vi "Wavelength Meter Control Panel (No Objects).vi"(8 "error in (no error)":errorcluster) -> (0 "error out":errorcluster)   [LabVIEW 2012]
doc: "(Dynamic) A user-level application that simulates the physical front panel of the Instrument. Provide the user with buttons to manually control features of the instrument, and provide indicators of its current state."
uses:
  HighFinesse WS5/Variable Typedefs.llb/Exposure Mode.ctl
  HighFinesse WS5/Control typedefs.llb/Measurement Mode.ctl
  HighFinesse WS5/HighFinesse WS5.lvlib
panel:
  in  "Cluster In":T3={"Exp Range Min"=0, "Exp Range Max"=0, "exposure mode"=enum."manual", "operation (meas. mode)"=enum."Measurement mode", "Exposure (ms)"=0, "Quiet Errors?"=FALSE, "Error Status"={"status"=FALSE, "code"=0, "source"=""}}
  out "Ready":bool
  out "Exposure (ms)":u16
  in  "Exposure Mode":T1
  in  "stop":bool
  in  "Read":bool
  in  "Set Exposure (ms)":u16
  out "Wavelength":dbl
  in  "Copy Actual to set":bool
  in  "Populate Fields with member data":bool
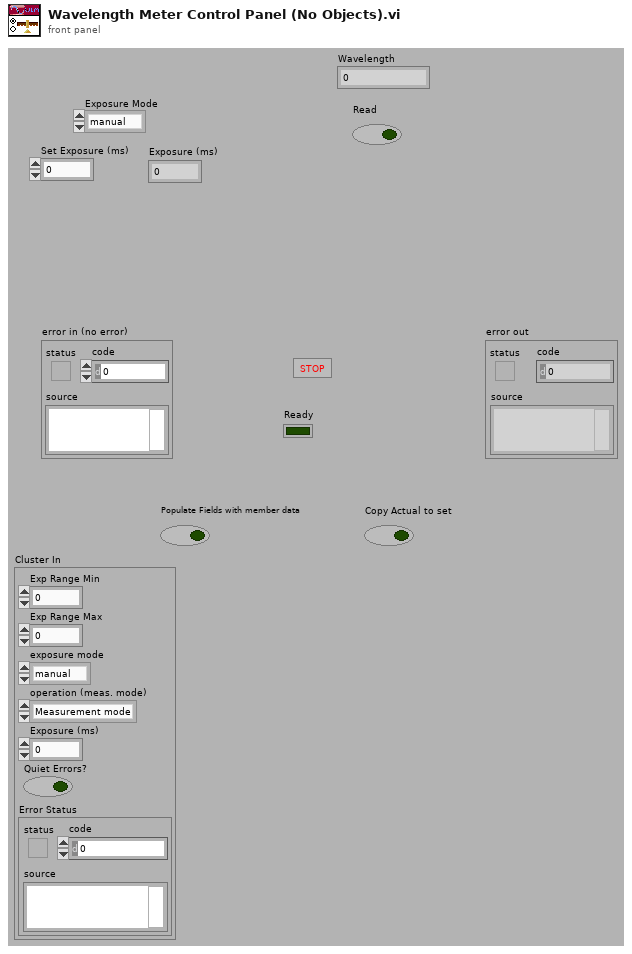
[diagram p1: front panel]
types:
  T1 = typedef "HighFinesse WS5.lvlib/Exposure Mode.ctl" = enum16{"manual", "automatic"}
  T2 = typedef "HighFinesse WS5.lvlib/Measurement Mode.ctl" = enum16{"Measurement off", "Adjustment mode", "Measurement mode"}
  T3 = cluster{"Exp Range Min":u32, "Exp Range Max":u32, "exposure mode":T1, "operation (meas. mode)":T2, "Exposure (ms)":u16, "Quiet Errors?":bool, "Error Status":errorcluster}
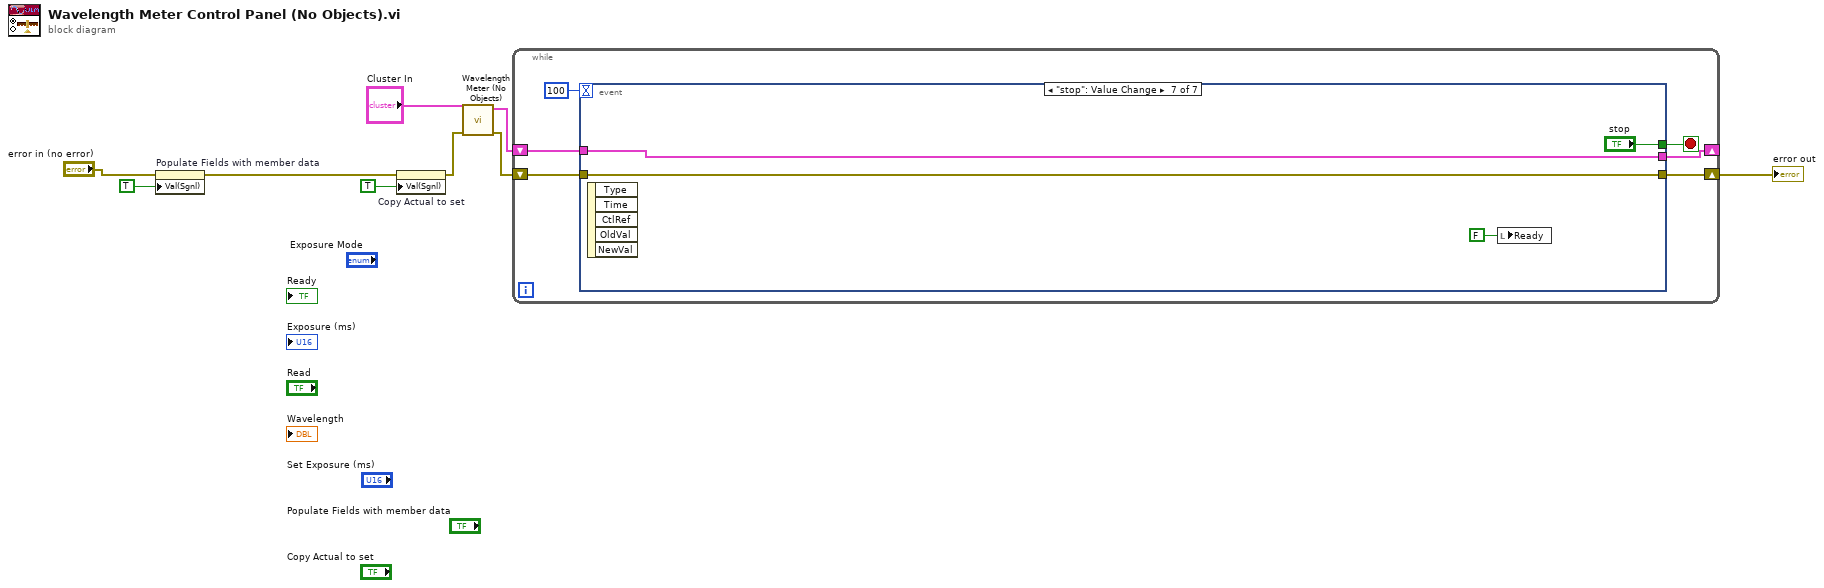
[diagram p0: block diagram]
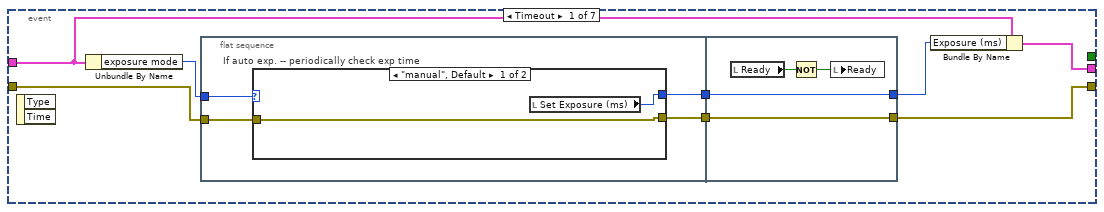
[diagram p2: hidden frame]
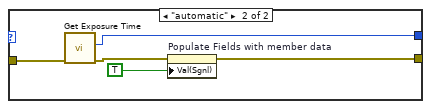
[diagram p3: hidden frame]
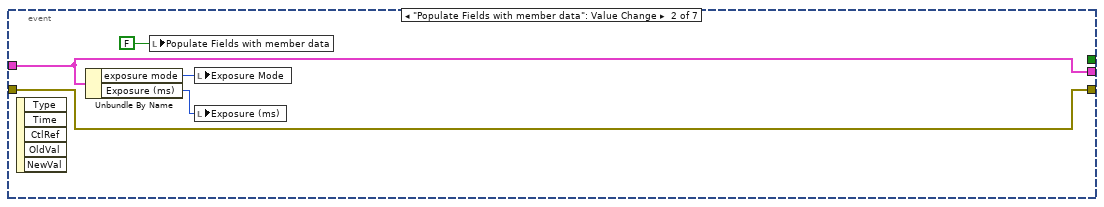
[diagram p4: hidden frame]
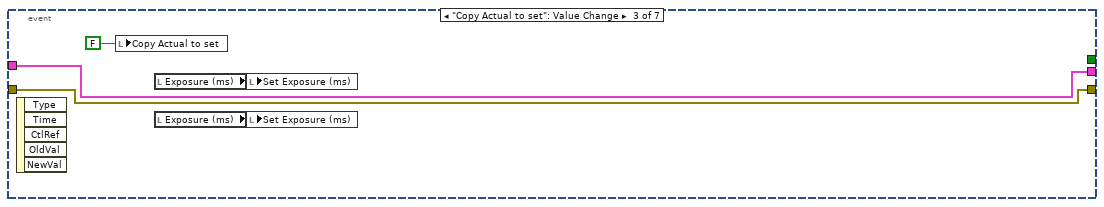
[diagram p5: hidden frame]
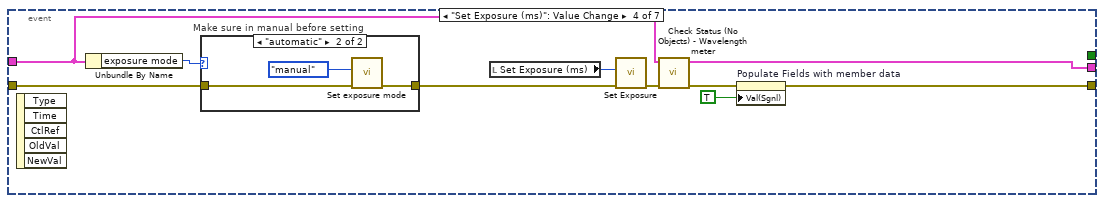
[diagram p6: hidden frame]
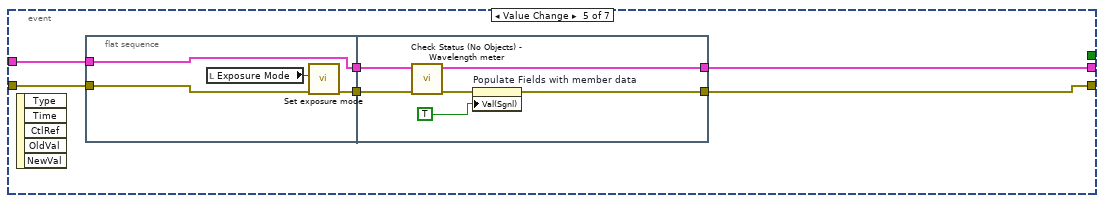
[diagram p8: hidden frame]
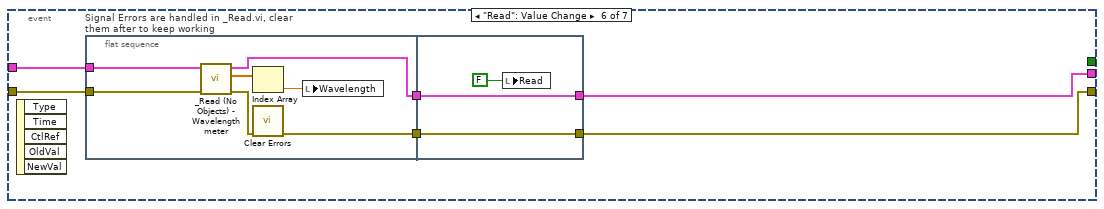
[diagram p9: hidden frame]
diagram:
  n1 = property on="Populate Fields with member data" class="Bool (strict)"(error in="error in (no error)", "Val(Sgnl)"=TRUE ("Value (Signaling)")) -> (error out=w7:errorcluster)  [unwired: 1 in, 1 out]
  n2 = property on="Copy Actual to set" class="Bool (strict)"(error in=w7, "Val(Sgnl)"=TRUE ("Value (Signaling)")) -> (error out=w4:errorcluster)  [unwired: 1 in, 1 out]
  n3 = call "Wavelength Meter (No Objects).vi"("error in (no error)"=w4, "Cluster In"="Cluster In") -> ("error out"=w3:errorcluster, "Cluster Out"=w2:T3)  [unwired: 8 in]
  n4 = while {
    shift-right: [w14] -> _
    shift-left: w2 -> [w15]
    shift-right: [w12] -> w5
    shift-left: w3 -> [w13]
    stop <- w11 stop-if-true
    n5 = event shown="[6] \"stop\": Value Change" {
      selector: _ -> [_ _ _ _ _ _ _]
      dyn-events: _ -> [_ _ _ _ _ _ _]
      timeout: 100 -> [_ _ _ _ _ _ _]
      tunnel: w15 -> [w20 w42 w48 w49 w65 w84 w97]
      tunnel: [w18 w42 w48 w53 w63 w82 w97] -> w14
      tunnel: [w21 w43 w47 w51 w66 w81 w96] -> w12
      tunnel: w13 -> [w22 w43 w47 w58 w68 w83 w96]
      tunnel: [_ _ _ _ _ _ "stop"] -> w11
      event Timeout {
        n6 = event-data() -> ()  [unwired: 1 in, 2 out]
        n7 = Unbundle By Name(w20) -> ("exposure mode"=w23:T1)
        n8 = flat-sequence {
          tunnel: w23 -> [w27]
          tunnel: w22 -> [w26]
          tunnel: [w25] -> w17
          tunnel: [w24] -> w16
          tunnel: [w38] -> w19
          tunnel: [w35] -> w21
          tunnel: w17 -> [w35]
          tunnel: w16 -> [w38]
          frame #0 {
            n9 = case "If auto exp. -- periodically check exp time" shown="\"manual\", Default" w27 {
              tunnel: w26 -> [w29 w34]
              tunnel: [w29 w30] -> w25
              tunnel: [w28 w33] -> w24
              frame "manual", Default {
                n10 = local read "Set Exposure (ms)"() -> (w28:u16)
              }
              frame "automatic" {
                n11 = call "Get Exposure Time.vi"("error in (no error)"=w34) -> ("error out"=w31:errorcluster, "Exposure (ms)"=w33:u16)  [unwired: 9 in]
                n12 = property on="Populate Fields with member data" class="Bool (strict)"(error in=w31, "Val(Sgnl)"=TRUE ("Value (Signaling)")) -> (error out=w30:errorcluster)  [unwired: 1 in, 1 out]
              }
            }
          }
          frame #1 {
            n13 = local read "Ready"() -> (w37:bool)
            n14 = Not(x=w37) -> (.not. x?=w36:bool)
            n15 = local write "Ready"(w36) -> ()
          }
        }
        n16 = Bundle By Name(cluster=w20, "Exposure (ms)"=w19) -> (w18:T3)
      }
      event "Populate Fields with member data": Value Change {
        n17 = event-data() -> ()  [unwired: 1 in, 5 out]
        n18 = Unbundle By Name(w42) -> ("exposure mode"=w41:T1, "Exposure (ms)"=w40:u16)
        n19 = local write "Populate Fields with member data"(FALSE ("Populate Fields with member data")) -> ()
        n20 = local write "Exposure Mode"(w41) -> ()
        n21 = local write "Exposure (ms)"(w40) -> ()
      }
      event "Copy Actual to set": Value Change {
        n22 = event-data() -> ()  [unwired: 1 in, 5 out]
        n23 = local write "Copy Actual to set"(FALSE ("Copy Actual to set")) -> ()
        n24 = local read "Exposure (ms)"() -> (w45:u16)
        n25 = local read "Exposure (ms)"() -> (w46:u16)
        n26 = local write "Set Exposure (ms)"(w45) -> ()
        n27 = local write "Set Exposure (ms)"(w46) -> ()
      }
      event "Set Exposure (ms)": Value Change {
        n28 = event-data() -> ()  [unwired: 1 in, 5 out]
        n29 = Unbundle By Name(w49) -> ("exposure mode"=w57:T1)
        n30 = case "Make sure in manual before setting" shown="\"automatic\"" w57 {
          tunnel: w58 -> [w59 w62]
          tunnel: [w59 w61] -> w56
          frame "manual", Default {
          }
          frame "automatic" {
            n31 = call "Set exposure mode.vi"("error in (no error)"=w62, "exposure mode"=Exposure_Mode."manual") -> ("error out"=w61:errorcluster)  [unwired: 8 in, 1 out]
          }
        }
        n32 = local read "Set Exposure (ms)"() -> (w55:u16)
        n33 = call "Set Exposure.vi"("error in (no error)"=w56, "Exposure (ms)"=w55) -> ("error out"=w54:errorcluster)  [unwired: 9 in]
        n34 = call "Check Status (No Objects) - Wavelength meter.vi"("error in (no error)"=w54, "Cluster In"=w49) -> ("error out"=w52:errorcluster, "Cluster Out"=w53:T3)  [unwired: 6 in, 2 out]
        n35 = property on="Populate Fields with member data" class="Bool (strict)"(error in=w52, "Val(Sgnl)"=TRUE ("Value (Signaling)")) -> (error out=w51:errorcluster)  [unwired: 1 in, 1 out]
      }
      event Value Change {
        n36 = event-data() -> ()  [unwired: 1 in, 5 out]
        n37 = flat-sequence {
          tunnel: w68 -> [w72]
          tunnel: [w70] -> w67
          tunnel: w65 -> [w69]
          tunnel: [w69] -> w64
          tunnel: w67 -> [w78]
          tunnel: [w76] -> w66
          tunnel: w64 -> [w73]
          tunnel: [w75] -> w63
          frame #0 {
            n38 = local read "Exposure Mode"() -> (w71:T1)
            n39 = call "Set exposure mode.vi"("error in (no error)"=w72, "exposure mode"=w71) -> ("error out"=w70:errorcluster)  [unwired: 8 in, 1 out]
          }
          frame #1 {
            n40 = call "Check Status (No Objects) - Wavelength meter.vi"("error in (no error)"=w78, "Cluster In"=w73) -> ("error out"=w77:errorcluster, "Cluster Out"=w75:T3)  [unwired: 6 in, 2 out]
            n41 = property on="Populate Fields with member data" class="Bool (strict)"(error in=w77, "Val(Sgnl)"=TRUE ("Value (Signaling)")) -> (error out=w76:errorcluster)  [unwired: 1 in, 1 out]
          }
        }
      }
      event "Read": Value Change {
        n42 = event-data() -> ()  [unwired: 1 in, 5 out]
        n43 = flat-sequence "Signal Errors are handled in _Read.vi, clear them after to keep working" {
          tunnel: w84 -> [w85]
          tunnel: w83 -> [w91]
          tunnel: [w88] -> w80
          tunnel: [w86] -> w79
          tunnel: [w93] -> w81
          tunnel: [w94] -> w82
          tunnel: w80 -> [w94]
          tunnel: w79 -> [w93]
          frame #0 {
            n44 = call "_Read (No Objects) - Wavelength meter.vi"("error in (no error)"=w91, "Cluster In"=w85) -> ("error out"=w87:errorcluster, "4 Data Points"=w90:dbl[], "Cluster Out"=w88:T3)  [unwired: 7 in]
            n45 = Index Array(array=w90) -> (element=w89:dbl)  [unwired: 1 in]
            n46 = call <vilib>:"Clear Errors.vi"("error in (no error)"=w87) -> ("error out"=w86:errorcluster)  [unwired: 6 in]
            n47 = local write "Wavelength"(w89) -> ()
          }
          frame #1 {
            n48 = local write "Read"(FALSE ("Read")) -> ()
          }
        }
      }
      event "stop": Value Change {
        n49 = event-data() -> ()  [unwired: 1 in, 5 out]
        n50 = local write "Ready"(FALSE ("Ready")) -> ()
      }
    }
  }
  "error out" <- w5
